vi "T'触发器(2分频).vi"(2 "error in (no error)":errorcluster caption="错误输入（无错误）", 3 "CP":bool) -> (0 "error out":errorcluster caption="错误输出", 1 "Q":bool)   [LabVIEW 2012, in "触发器.lvlib"]
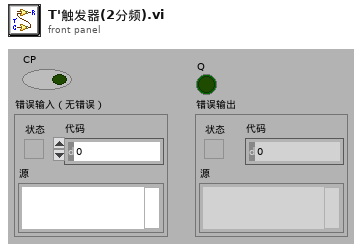
[diagram p1: front panel]
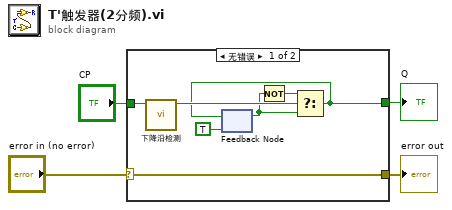
[diagram p0: block diagram]
diagram:
  n1 = case shown="无错误" "error in (no error)" {
    selector: "error in (no error)" -> [w7 w12]
    tunnel: [w7 w12] -> w3
    tunnel: "CP" -> [w6 _]
    tunnel: [w5 _] -> w1
    frame No Error {
      n2 = call "下降沿检测.vi"("input"=w6) -> ("output"=w11:bool)  [unwired: 9 in, 1 out]
      n3 = feedback #1(TRUE) -> (w9:bool)
      n4 = Not(x=w9) -> (.not. x?=w10:bool)
      n5 = Select(t=w10, s=w11, f=w9) -> (s? t:f=w5:bool)
      n6 = feedback-in #1(w5) -> ()
    }
    frame Error {
    }
  }
  "error out" <- w3
  "Q" <- w1
